vi "Fade-in UI.vi"(8 "error in":errorcluster, 11 "This VI":refnum<vi>) -> (0 "error out":errorcluster)   [LabVIEW 2020, in "UI Manager.lvlib"]
doc: "____\nHAMPEL SOFTWARE ENGINEERING v2.6.0 (2023-12-19 10:54)"
uses:
  UI Manager.lvlib
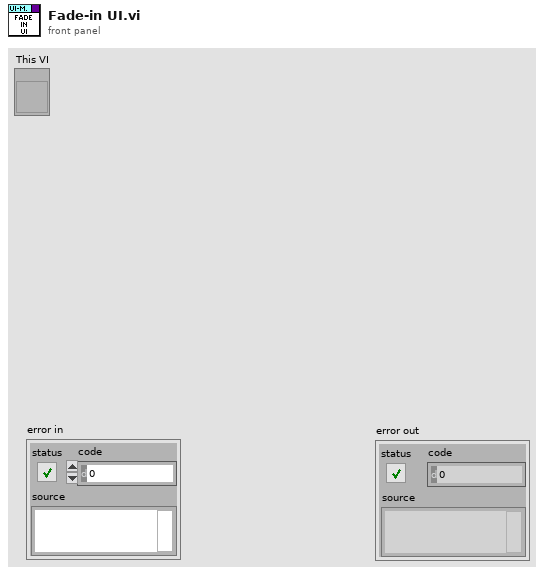
[diagram p1: front panel]
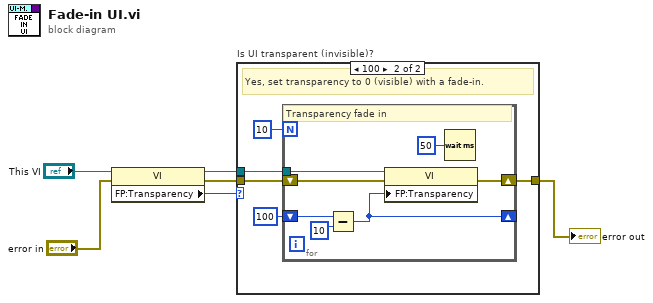
[diagram p0: block diagram]
diagram:
  n1 = property class="VI"(reference="This VI", error in="error in") -> (reference out=w5:refnum<vi>, error out=w4:errorcluster, "FP:Transparency"=w1:u8)
  n2 = case "Is UI transparent (invisible)?" shown="100" w1 {
    tunnel: w5 -> [_ w10]
    tunnel: w4 -> [w7 w9]
    tunnel: [w7 w8] -> w3
    frame 0, Default {
      # "No. do nothing."
    }
    frame 100 {
      # "Yes, set transparency to 0 (visible) with a fade-in."
      n3 = for {
        N: 10 -> [_]
        tunnel: w10 -> [w17]
        shift-right: [w18] -> w8
        shift-left: w9 -> [w19]
        shift-right: [w13] -> _
        shift-left: u8 100 ("Front Panel Window:Transparency") -> [w15]
        # "Transparency fade in"
        n4 = Subtract(x=w15, y=u8 10) -> (x-y=w13:u8)
        n5 = property class="VI"(reference=w17, error in=w19, "FP:Transparency"=w13) -> (error out=w18:errorcluster)  [unwired: 1 out]
        n6 = Wait (ms)(milliseconds to wait=u32 50) -> ()  [unwired: 1 out]
      }
    }
  }
  "error out" <- w3
